vi "添加数据.vi"(6 "测试数据输入":dbl[][](array[numeric]), 8 "错误输入（无错误）":errorcluster, 10 "数据":variant) -> (0 "错误输出":errorcluster, 4 "测试数据输出":dbl[][](array[numeric]))   [LabVIEW 2021]
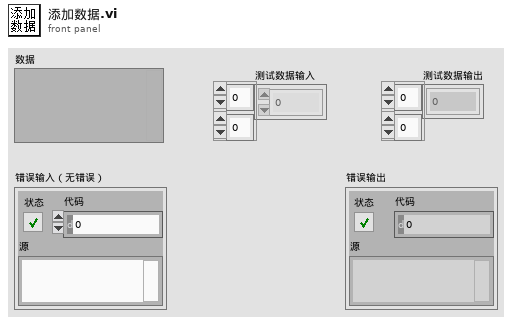
[diagram p1: front panel]
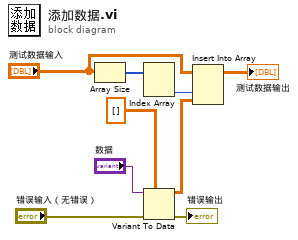
[diagram p0: block diagram]
diagram:
  n1 = Array Size(array="测试数据输入") -> (size(s)=w8:i32[])
  n2 = Index Array(array=w8) -> (element #2=w7:i32)  [unwired: 2 in, 1 out]
  n3 = Variant To Data(error in="错误输入（无错误）", type=dbl[][] [] ("测试数据"), Variant="数据") -> (data=w5:dbl[][], error out=→"错误输出":errorcluster)
  n4 = Insert Into Array(array="测试数据输入", index (col)=w7, new element=w5) -> (→"测试数据输出":dbl[][])  [unwired: 1 in]
